vi "Lab Panel V5.25.vi"() -> ()   [LabVIEW 2017] (continued)
                        n1485 = stacked-sequence {
                          tunnel: w2788 -> [w2791 _]
                          tunnel: w2787 -> [_ w2796]
                          tunnel: w2786 -> [w2789 _]
                          frame #0 {
                            n1486 = Build Array("T-RISE") -> (w2793:string[])
                            n1487 = Build Array(w2791) -> (w2792:dbl[])
                            n1488 = TDMS Write(0:w2789, 5:"TEST PASS", 7:w2793, 9:w2792) -> (15:w2795:errorcluster)  [unwired: 2 in, 3 out]
                            n1489 = local write "data file error"(w2795) -> ()
                          }
                          frame #1 {
                            n1490 = Bundle(cluster=w2796, "STATUS"="T-RISE PASS") -> (w2798:T4)  [unwired: 2 in]
                            n1491 = local write "RESULT LAB05-1"(TRUE) -> ()
                            n1492 = local write "DISP LAB05-1"(w2798) -> ()
                          }
                        }
                      }
                      frame False {
                      }
                    }
                  }
                }
              }
              frame #9 {
                # "LAB05-2"
                n1493 = Equal?(x=w2801, y=2) -> (x = y?=w2804:bool)
                n1494 = local read "DISP LAB05-2"() -> (w2806:T4)
                n1495 = Unbundle(w2806) -> ("STATUS"=w2807:string)  [unwired: 2 out]
                n1496 = Equal?(x=w2807, y="RUN") -> (x = y?=w2803:bool)
                n1497 = And(x=w2803, y=w2804) -> (x .and. y?=w2802:bool)
                n1498 = case shown="True" w2802 {
                  tunnel: w2806 -> [_ w2810]
                  tunnel: w2800 -> [_ w2813]
                  frame False {
                  }
                  frame True {
                    n1499 = local read "SET LAB05-2"() -> (w2812:T5)
                    n1500 = local read "TDMS LAB05-2"() -> (w2809:refnum<k34>)
                    n1501 = Unbundle(w2810) -> ("CYCLE"=w2814:dbl)  [unwired: 2 out]
                    n1502 = Unbundle(w2812) -> ("T-RISE mins"=w2811:dbl)  [unwired: 4 out]
                    n1503 = Greater Or Equal?(x=w2814, y=w2813) -> (x >= y?=w2815:bool)
                    n1504 = case shown="True" w2815 {
                      tunnel: w2811 -> [w2818 _]
                      tunnel: w2810 -> [w2817 _]
                      tunnel: w2809 -> [w2816 _]
                      frame True {
                        n1505 = stacked-sequence {
                          tunnel: w2818 -> [w2821 _]
                          tunnel: w2817 -> [_ w2826]
                          tunnel: w2816 -> [w2819 _]
                          frame #0 {
                            n1506 = Build Array("T-RISE") -> (w2823:string[])
                            n1507 = Build Array(w2821) -> (w2822:dbl[])
                            n1508 = TDMS Write(0:w2819, 5:"TEST PASS", 7:w2823, 9:w2822) -> (15:w2825:errorcluster)  [unwired: 2 in, 3 out]
                            n1509 = local write "data file error"(w2825) -> ()
                          }
                          frame #1 {
                            n1510 = Bundle(cluster=w2826, "STATUS"="T-RISE PASS") -> (w2828:T4)  [unwired: 2 in]
                            n1511 = local write "RESULT LAB05-2"(TRUE) -> ()
                            n1512 = local write "DISP LAB05-2"(w2828) -> ()
                          }
                        }
                      }
                      frame False {
                      }
                    }
                  }
                }
              }
            }
          }
          frame #6 {
            # "end test & close test files"
            n1513 = local read "MAIL SETTINGS"() -> (w2834:T7)
            n1514 = Unbundle(w2834) -> ("OUT SERVER ADDRESS"=w2833:string, "FROM ACCOUNT"=w2832:string)  [unwired: 5 out]
            n1515 = stacked-sequence {
              tunnel: w2844 -> [_ _ _ _ _ _ _ _ _ _]
              tunnel: w2845 -> [_ _ _ _ _ _ _ _ _ _]
              tunnel: w2843 -> [_ _ _ _ _ _ _ _ _ _]
              tunnel: w2842 -> [_ _ _ _ _ _ _ _ _ _]
              tunnel: w2841 -> [_ _ _ _ _ _ _ _ _ _]
              tunnel: w2840 -> [_ _ _ _ _ _ _ _ _ _]
              tunnel: w2839 -> [_ _ _ _ _ _ _ _ _ _]
              tunnel: w2838 -> [_ _ _ _ _ _ _ _ _ _]
              tunnel: w2837 -> [_ _ _ _ _ _ _ _ _ _]
              tunnel: w2836 -> [_ _ _ _ _ _ _ _ _ _]
              tunnel: w2833 -> [w2849 w2901 w2949 w2996 w3043 w3090 w3137 w3184 w3231 w3278]
              tunnel: w2832 -> [w2848 w2900 w2948 w2995 w3042 w3089 w3136 w3183 w3230 w3277]
              tunnel: "Mail Test File To:" -> [w2847 w2899 w2947 w2994 w3041 w3088 w3135 w3182 w3229 w3276]
              tunnel: "Mail Test Fail" -> [w2846 w2898 w2946 w2993 w3040 w3087 w3134 w3181 w3228 w3275]
              frame #0 {
                # "LAB01-1"
                n1516 = local read "DISP LAB01-1"() -> (w2853:T4)
                n1517 = local read "run lab01-1"() -> (w2850:bool)
                n1518 = local read "TDMS LAB01-1"() -> (w2851:refnum<k34>)
                n1519 = Unbundle(w2853) -> ("CYCLE"=w2854:dbl, "STATUS"=w2852:string)  [unwired: 1 out]
                n1520 = case shown="True" w2850 {
                  tunnel: w2854 -> [_ w2860]
                  tunnel: w2853 -> [_ w2862]
                  tunnel: w2852 -> [_ w2859]
                  tunnel: w2851 -> [_ w2861]
                  tunnel: w2849 -> [_ w2858]
                  tunnel: w2848 -> [_ w2857]
                  tunnel: w2847 -> [_ w2856]
                  tunnel: w2846 -> [_ w2855]
                  frame False {
                  }
                  frame True {
                    n1521 = Not Equal?(x=w2859, y="RUN") -> (x != y?=w2863:bool)
                    n1522 = Greater?(x=w2860, y=2.0) -> (0:w2865:bool)
                    n1523 = And(x=w2865, y=w2863) -> (x .and. y?=w2864:bool)
                    n1524 = case shown="True" w2864 {
                      tunnel: w2862 -> [_ w2875]
                      tunnel: w2861 -> [_ w2874]
                      tunnel: w2860 -> [_ w2873]
                      tunnel: w2859 -> [_ w2872]
                      tunnel: w2858 -> [_ w2871]
                      tunnel: w2857 -> [_ w2870]
                      tunnel: w2856 -> [_ w2869]
                      tunnel: w2855 -> [_ w2868]
                      frame False {
                      }
                      frame True {
                        n1525 = stacked-sequence {
                          tunnel: w2875 -> [w2879 _ _]
                          tunnel: w2874 -> [_ w2881 _]
                          tunnel: w2873 -> [_ _ _]
                          tunnel: w2872 -> [_ _ w2887]
                          tunnel: w2871 -> [_ _ w2886]
                          tunnel: w2870 -> [_ _ w2885]
                          tunnel: w2869 -> [_ _ w2884]
                          tunnel: w2868 -> [_ _ w2883]
                          frame #0 {
                            w2876 = FALSE
                            n1526 = local write "mail control"("END") -> ()
                            n1527 = Bundle(cluster=w2879) -> (w2878:T4)  [unwired: 3 in]
                            n1528 = local write "DISP LAB01-1"(w2878) -> ()
                            n1529 = local write "O/I  LAB01-1"(w2876) -> ()
                            n1530 = local write "run lab01-1"(w2876) -> ()
                            n1531 = local write "RUN LAB01-1"(w2876) -> ()
                          }
                          frame #1 {
                            n1532 = TDMS Close(11:w2881) -> (0:w2880:errorcluster)  [unwired: 1 in, 1 out]
                            n1533 = local write "data file error"(w2880) -> ()
                          }
                          frame #2 {
                            n1534 = stacked-sequence {
                              tunnel: "LAB01-1" -> [w2889 w2891 _]
                              tunnel: w2887 -> [_ w2897 _]
                              tunnel: w2886 -> [_ w2896 _]
                              tunnel: w2885 -> [_ w2895 _]
                              tunnel: w2884 -> [_ w2894 _]
                              tunnel: w2883 -> [_ w2893 _]
                              frame #0 {
                                n1535 = call "sub vi - defrag tdms v1.vi"("panel id"=w2889) -> ("error out"=w2888:errorcluster)  [unwired: 10 in]
                                n1536 = local write "data file error"(w2888) -> ()
                              }
                              frame #1 {
                                n1537 = Bundle("STATUS"=w2897, "OUT SERVER ADDRESS"=w2896, "FROM ACCOUNT"=w2895, "Mail Test File To:"=w2894, "Mail Test Fail"=w2893) -> (w2890:T26)  [unwired: 1 in]
                                n1538 = call "Save data file (pass-fail) v5.vi"("Input Cluster"=w2890, "panel id"=w2891) -> ("network file save error"=w2892:errorcluster)  [unwired: 8 in, 1 out]
                                n1539 = local write "data file error"(w2892) -> ()
                              }
                              frame #2 {
                              }
                            }
                          }
                        }
                      }
                    }
                  }
                }
              }
              frame #1 {
                # "LAB01-2"
                n1540 = local read "run lab01-2"() -> (w2902:bool)
                n1541 = case shown="True" w2902 {
                  tunnel: w2901 -> [_ w2906]
                  tunnel: w2900 -> [_ w2905]
                  tunnel: w2899 -> [_ w2904]
                  tunnel: w2898 -> [_ w2903]
                  frame False {
                  }
                  frame True {
                    n1542 = local read "DISP LAB01-2"() -> (w2914:T4)
                    n1543 = local read "TDMS LAB01-2"() -> (w2913:refnum<k34>)
                    n1544 = Unbundle(w2914) -> ("CYCLE"=w2908:dbl, "STATUS"=w2907:string)  [unwired: 1 out]
                    n1545 = Not Equal?(x=w2907, y="RUN") -> (x != y?=w2910:bool)
                    n1546 = Greater?(x=w2908, y=2.0) -> (0:w2911:bool)
                    n1547 = And(x=w2911, y=w2910) -> (x .and. y?=w2909:bool)
                    n1548 = case shown="True" w2909 {
                      tunnel: w2914 -> [_ w2923]
                      tunnel: w2913 -> [_ w2922]
                      tunnel: w2908 -> [_ w2921]
                      tunnel: w2907 -> [_ w2920]
                      tunnel: w2906 -> [_ w2919]
                      tunnel: w2905 -> [_ w2918]
                      tunnel: w2904 -> [_ w2917]
                      tunnel: w2903 -> [_ w2916]
                      frame False {
                      }
                      frame True {
                        n1549 = stacked-sequence {
                          tunnel: w2923 -> [w2926 _ _]
                          tunnel: w2922 -> [_ w2928 _]
                          tunnel: w2921 -> [_ _ _]
                          tunnel: w2920 -> [_ _ w2934]
                          tunnel: w2919 -> [_ _ w2933]
                          tunnel: w2918 -> [_ _ w2932]
                          tunnel: w2917 -> [_ _ w2931]
                          tunnel: w2916 -> [_ _ w2930]
                          frame #0 {
                            w2924 = FALSE
                            n1550 = local write "mail control"("END") -> ()
                            n1551 = Bundle(cluster=w2926) -> (w2927:T4)  [unwired: 3 in]
                            n1552 = local write "RUN LAB01-2"(w2924) -> ()
                            n1553 = local write "run lab01-2"(w2924) -> ()
                            n1554 = local write "O/I  LAB01-2"(w2924) -> ()
                            n1555 = local write "DISP LAB01-2"(w2927) -> ()
                          }
                          frame #1 {
                            n1556 = TDMS Close(11:w2928) -> (0:w2929:errorcluster)  [unwired: 1 in, 1 out]
                            n1557 = local write "data file error"(w2929) -> ()
                          }
                          frame #2 {
                            n1558 = stacked-sequence {
                              tunnel: "LAB01-2" -> [w2937 w2938]
                              tunnel: w2934 -> [_ w2943]
                              tunnel: w2933 -> [_ w2942]
                              tunnel: w2932 -> [_ w2941]
                              tunnel: w2931 -> [_ w2940]
                              tunnel: w2930 -> [_ w2939]
                              frame #0 {
                                n1559 = call "sub vi - defrag tdms v1.vi"("panel id"=w2937) -> ("error out"=w2936:errorcluster)  [unwired: 10 in]
                                n1560 = local write "data file error"(w2936) -> ()
                              }
                              frame #1 {
                                n1561 = Bundle("STATUS"=w2943, "OUT SERVER ADDRESS"=w2942, "FROM ACCOUNT"=w2941, "Mail Test File To:"=w2940, "Mail Test Fail"=w2939) -> (w2945:T26)  [unwired: 1 in]
                                n1562 = call "Save data file (pass-fail) v5.vi"("Input Cluster"=w2945, "panel id"=w2938) -> ("network file save error"=w2944:errorcluster)  [unwired: 8 in, 1 out]
                                n1563 = local write "data file error"(w2944) -> ()
                              }
                            }
                          }
                        }
                      }
                    }
                  }
                }
              }
              frame #2 {
                # "LAB02-1"
                n1564 = local read "run lab02-1"() -> (w2950:bool)
                n1565 = case shown="True" w2950 {
                  tunnel: w2949 -> [_ w2954]
                  tunnel: w2948 -> [_ w2953]
                  tunnel: w2947 -> [_ w2952]
                  tunnel: w2946 -> [_ w2951]
                  frame False {
                  }
                  frame True {
                    n1566 = local read "DISP LAB02-1"() -> (w2962:T4)
                    n1567 = Unbundle(w2962) -> ("CYCLE"=w2958:dbl, "STATUS"=w2955:string)  [unwired: 1 out]
                    n1568 = local read "TDMS LAB02-1"() -> (w2961:refnum<k34>)
                    n1569 = Not Equal?(x=w2955, y="RUN") -> (x != y?=w2957:bool)
                    n1570 = Greater?(x=w2958, y=2.0) -> (0:w2959:bool)
                    n1571 = And(x=w2959, y=w2957) -> (x .and. y?=w2956:bool)
                    n1572 = case shown="True" w2956 {
                      tunnel: w2962 -> [_ w2970]
                      tunnel: w2961 -> [_ w2969]
                      tunnel: w2955 -> [_ w2968]
                      tunnel: w2954 -> [_ w2967]
                      tunnel: w2953 -> [_ w2966]
                      tunnel: w2952 -> [_ w2965]
                      tunnel: w2951 -> [_ w2964]
                      frame False {
                      }
                      frame True {
                        n1573 = stacked-sequence {
                          tunnel: w2970 -> [w2973 _ _]
                          tunnel: w2969 -> [_ w2975 _]
                          tunnel: w2968 -> [_ _ w2981]
                          tunnel: w2967 -> [_ _ w2980]
                          tunnel: w2966 -> [_ _ w2979]
                          tunnel: w2965 -> [_ _ w2978]
                          tunnel: w2964 -> [_ _ w2977]
                          frame #0 {
                            w2971 = FALSE
                            n1574 = local write "mail control"("END") -> ()
                            n1575 = Bundle(cluster=w2973) -> (w2974:T4)  [unwired: 3 in]
                            n1576 = local write "O/I  LAB02-1"(w2971) -> ()
                            n1577 = local write "RUN LAB02-1"(w2971) -> ()
                            n1578 = local write "run lab02-1"(w2971) -> ()
                            n1579 = local write "DISP LAB02-1"(w2974) -> ()
                          }
                          frame #1 {
                            n1580 = TDMS Close(11:w2975) -> (0:w2976:errorcluster)  [unwired: 1 in, 1 out]
                            n1581 = local write "data file error"(w2976) -> ()
                          }
                          frame #2 {
                            n1582 = stacked-sequence {
                              tunnel: "LAB02-1" -> [w2984 w2991]
                              tunnel: w2981 -> [_ w2989]
                              tunnel: w2980 -> [_ w2988]
                              tunnel: w2979 -> [_ w2987]
                              tunnel: w2978 -> [_ w2986]
                              tunnel: w2977 -> [_ w2985]
                              frame #0 {
                                n1583 = call "sub vi - defrag tdms v1.vi"("panel id"=w2984) -> ("error out"=w2983:errorcluster)  [unwired: 10 in]
                                n1584 = local write "data file error"(w2983) -> ()
                              }
                              frame #1 {
                                n1585 = Bundle("STATUS"=w2989, "OUT SERVER ADDRESS"=w2988, "FROM ACCOUNT"=w2987, "Mail Test File To:"=w2986, "Mail Test Fail"=w2985) -> (w2990:T26)  [unwired: 1 in]
                                n1586 = call "Save data file (pass-fail) v5.vi"("Input Cluster"=w2990, "panel id"=w2991) -> ("network file save error"=w2992:errorcluster)  [unwired: 8 in, 1 out]
                                n1587 = local write "data file error"(w2992) -> ()
                              }
                            }
                          }
                        }
                      }
                    }
                  }
                }
              }
              frame #3 {
                # "LAB02-2"
                n1588 = local read "run lab02-2"() -> (w2997:bool)
                n1589 = case shown="True" w2997 {
                  tunnel: w2996 -> [_ w3001]
                  tunnel: w2995 -> [_ w3000]
                  tunnel: w2994 -> [_ w2999]
                  tunnel: w2993 -> [_ w2998]
                  frame False {
                  }
                  frame True {
                    n1590 = local read "DISP LAB02-2"() -> (w3009:T4)
                    n1591 = local read "TDMS LAB02-2"() -> (w3008:refnum<k34>)
                    n1592 = Unbundle(w3009) -> ("CYCLE"=w3005:dbl, "STATUS"=w3002:string)  [unwired: 1 out]
                    n1593 = Not Equal?(x=w3002, y="RUN") -> (x != y?=w3004:bool)
                    n1594 = Greater?(x=w3005, y=2.0) -> (0:w3006:bool)
                    n1595 = And(x=w3006, y=w3004) -> (x .and. y?=w3003:bool)
                    n1596 = case shown="True" w3003 {
                      tunnel: w3009 -> [_ w3017]
                      tunnel: w3008 -> [_ w3016]
                      tunnel: w3002 -> [_ w3015]
                      tunnel: w3001 -> [_ w3014]
                      tunnel: w3000 -> [_ w3013]
                      tunnel: w2999 -> [_ w3012]
                      tunnel: w2998 -> [_ w3011]
                      frame False {
                      }
                      frame True {
                        n1597 = stacked-sequence {
                          tunnel: w3017 -> [w3020 _ _]
                          tunnel: w3016 -> [_ w3022 _]
                          tunnel: w3015 -> [_ _ w3028]
                          tunnel: w3014 -> [_ _ w3027]
                          tunnel: w3013 -> [_ _ w3026]
                          tunnel: w3012 -> [_ _ w3025]
                          tunnel: w3011 -> [_ _ w3024]
                          frame #0 {
                            w3018 = FALSE
                            n1598 = local write "mail control"("END") -> ()
                            n1599 = Bundle(cluster=w3020) -> (w3021:T4)  [unwired: 3 in]
                            n1600 = local write "O/I  LAB02-2"(w3018) -> ()
                            n1601 = local write "run lab02-2"(w3018) -> ()
                            n1602 = local write "RUN LAB02-2"(w3018) -> ()
                            n1603 = local write "DISP LAB02-2"(w3021) -> ()
                          }
                          frame #1 {
                            n1604 = TDMS Close(11:w3022) -> (0:w3023:errorcluster)  [unwired: 1 in, 1 out]
                            n1605 = local write "data file error"(w3023) -> ()
                          }
                          frame #2 {
                            n1606 = stacked-sequence {
                              tunnel: "LAB02-2" -> [w3031 w3037]
                              tunnel: w3028 -> [_ w3036]
                              tunnel: w3027 -> [_ w3035]
                              tunnel: w3026 -> [_ w3034]
                              tunnel: w3025 -> [_ w3033]
                              tunnel: w3024 -> [_ w3032]
                              frame #0 {
                                n1607 = call "sub vi - defrag tdms v1.vi"("panel id"=w3031) -> ("error out"=w3030:errorcluster)  [unwired: 10 in]
                                n1608 = local write "data file error"(w3030) -> ()
                              }
                              frame #1 {
                                n1609 = Bundle("STATUS"=w3036, "OUT SERVER ADDRESS"=w3035, "FROM ACCOUNT"=w3034, "Mail Test File To:"=w3033, "Mail Test Fail"=w3032) -> (w3039:T26)  [unwired: 1 in]
                                n1610 = call "Save data file (pass-fail) v5.vi"("Input Cluster"=w3039, "panel id"=w3037) -> ("network file save error"=w3038:errorcluster)  [unwired: 8 in, 1 out]
                                n1611 = local write "data file error"(w3038) -> ()
                              }
                            }
                          }
                        }
                      }
                    }
                  }
                }
              }
              frame #4 {
                # "LAB03-1"
                n1612 = local read "run lab03-1"() -> (w3044:bool)
                n1613 = case shown="True" w3044 {
                  tunnel: w3043 -> [_ w3048]
                  tunnel: w3042 -> [_ w3047]
                  tunnel: w3041 -> [_ w3046]
                  tunnel: w3040 -> [_ w3045]
                  frame False {
                  }
                  frame True {
                    n1614 = local read "DISP LAB03-1"() -> (w3056:T4)
                    n1615 = local read "TDMS LAB03-1"() -> (w3055:refnum<k34>)
                    n1616 = Unbundle(w3056) -> ("CYCLE"=w3052:dbl, "STATUS"=w3049:string)  [unwired: 1 out]
                    n1617 = Not Equal?(x=w3049, y="RUN") -> (x != y?=w3051:bool)
                    n1618 = Greater?(x=w3052, y=2.0) -> (0:w3053:bool)
                    n1619 = And(x=w3053, y=w3051) -> (x .and. y?=w3050:bool)
                    n1620 = case shown="True" w3050 {
                      tunnel: w3056 -> [_ w3064]
                      tunnel: w3055 -> [_ w3063]
                      tunnel: w3049 -> [_ w3062]
                      tunnel: w3048 -> [_ w3061]
                      tunnel: w3047 -> [_ w3060]
                      tunnel: w3046 -> [_ w3059]
                      tunnel: w3045 -> [_ w3058]
                      frame False {
                      }
                      frame True {
                        n1621 = stacked-sequence {
                          tunnel: w3064 -> [w3067 _ _]
                          tunnel: w3063 -> [_ w3069 _]
                          tunnel: w3062 -> [_ _ w3075]
                          tunnel: w3061 -> [_ _ w3074]
                          tunnel: w3060 -> [_ _ w3073]
                          tunnel: w3059 -> [_ _ w3072]
                          tunnel: w3058 -> [_ _ w3071]
                          frame #0 {
                            w3065 = FALSE
                            n1622 = local write "mail control"("END") -> ()
                            n1623 = Bundle(cluster=w3067) -> (w3068:T4)  [unwired: 3 in]
                            n1624 = local write "O/I  LAB03-1"(w3065) -> ()
                            n1625 = local write "run lab03-1"(w3065) -> ()
                            n1626 = local write "RUN LAB03-1"(w3065) -> ()
                            n1627 = local write "DISP LAB03-1"(w3068) -> ()
                          }
                          frame #1 {
                            n1628 = TDMS Close(11:w3069) -> (0:w3070:errorcluster)  [unwired: 1 in, 1 out]
                            n1629 = local write "data file error"(w3070) -> ()
                          }
                          frame #2 {
                            n1630 = stacked-sequence {
                              tunnel: "LAB03-1" -> [w3078 w3084]
                              tunnel: w3075 -> [_ w3083]
                              tunnel: w3074 -> [_ w3082]
                              tunnel: w3073 -> [_ w3081]
                              tunnel: w3072 -> [_ w3080]
                              tunnel: w3071 -> [_ w3079]
                              frame #0 {
                                n1631 = call "sub vi - defrag tdms v1.vi"("panel id"=w3078) -> ("error out"=w3077:errorcluster)  [unwired: 10 in]
                                n1632 = local write "data file error"(w3077) -> ()
                              }
                              frame #1 {
                                n1633 = Bundle("STATUS"=w3083, "OUT SERVER ADDRESS"=w3082, "FROM ACCOUNT"=w3081, "Mail Test File To:"=w3080, "Mail Test Fail"=w3079) -> (w3086:T26)  [unwired: 1 in]
                                n1634 = call "Save data file (pass-fail) v5.vi"("Input Cluster"=w3086, "panel id"=w3084) -> ("network file save error"=w3085:errorcluster)  [unwired: 8 in, 1 out]
                                n1635 = local write "data file error"(w3085) -> ()
                              }
                            }
                          }
                        }
                      }
                    }
                  }
                }
              }
              frame #5 {
                # "LAB03-2"
                n1636 = local read "run lab03-2"() -> (w3091:bool)
                n1637 = case shown="True" w3091 {
                  tunnel: w3090 -> [_ w3095]
                  tunnel: w3089 -> [_ w3094]
                  tunnel: w3088 -> [_ w3093]
                  tunnel: w3087 -> [_ w3092]
                  frame False {
                  }
                  frame True {
                    n1638 = local read "DISP LAB03-2"() -> (w3103:T4)
                    n1639 = Unbundle(w3103) -> ("CYCLE"=w3099:dbl, "STATUS"=w3096:string)  [unwired: 1 out]
                    n1640 = local read "TDMS LAB03-2"() -> (w3102:refnum<k34>)
                    n1641 = Not Equal?(x=w3096, y="RUN") -> (x != y?=w3098:bool)
                    n1642 = Greater?(x=w3099, y=2.0) -> (0:w3100:bool)
                    n1643 = And(x=w3100, y=w3098) -> (x .and. y?=w3097:bool)
                    n1644 = case shown="True" w3097 {
                      tunnel: w3103 -> [_ w3111]
                      tunnel: w3102 -> [_ w3110]
                      tunnel: w3096 -> [_ w3109]
                      tunnel: w3095 -> [_ w3108]
                      tunnel: w3094 -> [_ w3107]
                      tunnel: w3093 -> [_ w3106]
                      tunnel: w3092 -> [_ w3105]
                      frame False {
                      }
                      frame True {
                        n1645 = stacked-sequence {
                          tunnel: w3111 -> [w3114 _ _]
                          tunnel: w3110 -> [_ w3116 _]
                          tunnel: w3109 -> [_ _ w3122]
                          tunnel: w3108 -> [_ _ w3121]
                          tunnel: w3107 -> [_ _ w3120]
                          tunnel: w3106 -> [_ _ w3119]
                          tunnel: w3105 -> [_ _ w3118]
                          frame #0 {
                            w3112 = FALSE
                            n1646 = local write "mail control"("END") -> ()
                            n1647 = Bundle(cluster=w3114) -> (w3115:T4)  [unwired: 3 in]
                            n1648 = local write "RUN LAB03-2"(w3112) -> ()
                            n1649 = local write "O/I  LAB03-2"(w3112) -> ()
                            n1650 = local write "DISP LAB03-2"(w3115) -> ()
                            n1651 = local write "run lab03-2"(w3112) -> ()
                          }
                          frame #1 {
                            n1652 = TDMS Close(11:w3116) -> (0:w3117:errorcluster)  [unwired: 1 in, 1 out]
                            n1653 = local write "data file error"(w3117) -> ()
                          }
                          frame #2 {
                            n1654 = stacked-sequence {
                              tunnel: "LAB03-2" -> [w3125 w3126]
                              tunnel: w3122 -> [_ w3131]
                              tunnel: w3121 -> [_ w3130]
                              tunnel: w3120 -> [_ w3129]
                              tunnel: w3119 -> [_ w3128]
                              tunnel: w3118 -> [_ w3127]
                              frame #0 {
                                n1655 = call "sub vi - defrag tdms v1.vi"("panel id"=w3125) -> ("error out"=w3124:errorcluster)  [unwired: 10 in]
                                n1656 = local write "data file error"(w3124) -> ()
                              }
                              frame #1 {
                                n1657 = Bundle("STATUS"=w3131, "OUT SERVER ADDRESS"=w3130, "FROM ACCOUNT"=w3129, "Mail Test File To:"=w3128, "Mail Test Fail"=w3127) -> (w3133:T26)  [unwired: 1 in]
                                n1658 = call "Save data file (pass-fail) v5.vi"("Input Cluster"=w3133, "panel id"=w3126) -> ("network file save error"=w3132:errorcluster)  [unwired: 8 in, 1 out]
                                n1659 = local write "data file error"(w3132) -> ()
                              }
                            }
                          }
                        }
                      }
                    }
                  }
                }
              }
              frame #6 {
                # "LAB04-1"
                n1660 = local read "run lab04-1"() -> (w3138:bool)
                n1661 = case shown="True" w3138 {
                  tunnel: w3137 -> [_ w3142]
                  tunnel: w3136 -> [_ w3141]
                  tunnel: w3135 -> [_ w3140]
                  tunnel: w3134 -> [_ w3139]
                  frame False {
                  }
                  frame True {
                    n1662 = local read "DISP LAB04-1"() -> (w3150:T4)
                    n1663 = Unbundle(w3150) -> ("CYCLE"=w3146:dbl, "STATUS"=w3143:string)  [unwired: 1 out]
                    n1664 = local read "TDMS LAB04-1"() -> (w3149:refnum<k34>)
                    n1665 = Not Equal?(x=w3143, y="RUN") -> (x != y?=w3145:bool)
                    n1666 = Greater?(x=w3146, y=2.0) -> (0:w3147:bool)
                    n1667 = And(x=w3147, y=w3145) -> (x .and. y?=w3144:bool)
                    n1668 = case shown="True" w3144 {
                      tunnel: w3150 -> [_ w3158]
                      tunnel: w3149 -> [_ w3157]
                      tunnel: w3143 -> [_ w3156]
                      tunnel: w3142 -> [_ w3155]
                      tunnel: w3141 -> [_ w3154]
                      tunnel: w3140 -> [_ w3153]
                      tunnel: w3139 -> [_ w3152]
                      frame False {
                      }
                      frame True {
                        n1669 = stacked-sequence {
                          tunnel: w3158 -> [w3161 _ _]
                          tunnel: w3157 -> [_ w3163 _]
                          tunnel: w3156 -> [_ _ w3169]
                          tunnel: w3155 -> [_ _ w3168]
                          tunnel: w3154 -> [_ _ w3167]
                          tunnel: w3153 -> [_ _ w3166]
                          tunnel: w3152 -> [_ _ w3165]
                          frame #0 {
                            w3159 = FALSE
                            n1670 = local write "mail control"("END") -> ()
                            n1671 = Bundle(cluster=w3161) -> (w3162:T4)  [unwired: 3 in]
                            n1672 = local write "RUN LAB04-1"(w3159) -> ()
                            n1673 = local write "O/I  LAB04-1"(w3159) -> ()
                            n1674 = local write "run lab04-1"(w3159) -> ()
                            n1675 = local write "DISP LAB04-1"(w3162) -> ()
                          }
                          frame #1 {
                            n1676 = TDMS Close(11:w3163) -> (0:w3164:errorcluster)  [unwired: 1 in, 1 out]
                            n1677 = local write "data file error"(w3164) -> ()
                          }
                          frame #2 {
                            n1678 = stacked-sequence {
                              tunnel: "LAB04-1" -> [w3172 w3173]
                              tunnel: w3169 -> [_ w3178]
                              tunnel: w3168 -> [_ w3177]
                              tunnel: w3167 -> [_ w3176]
                              tunnel: w3166 -> [_ w3175]
                              tunnel: w3165 -> [_ w3174]
                              frame #0 {
                                n1679 = call "sub vi - defrag tdms v1.vi"("panel id"=w3172) -> ("error out"=w3171:errorcluster)  [unwired: 10 in]
                                n1680 = local write "data file error"(w3171) -> ()
                              }
                              frame #1 {
                                n1681 = Bundle("STATUS"=w3178, "OUT SERVER ADDRESS"=w3177, "FROM ACCOUNT"=w3176, "Mail Test File To:"=w3175, "Mail Test Fail"=w3174) -> (w3180:T26)  [unwired: 1 in]
                                n1682 = call "Save data file (pass-fail) v5.vi"("Input Cluster"=w3180, "panel id"=w3173) -> ("network file save error"=w3179:errorcluster)  [unwired: 8 in, 1 out]
                                n1683 = local write "data file error"(w3179) -> ()
                              }
                            }
                          }
                        }
                      }
                    }
                  }
                }
              }
              frame #7 {
                # "LAB04-2"
                n1684 = local read "run lab04-2"() -> (w3185:bool)
                n1685 = case shown="True" w3185 {
                  tunnel: w3184 -> [_ w3189]
                  tunnel: w3183 -> [_ w3188]
                  tunnel: w3182 -> [_ w3187]
                  tunnel: w3181 -> [_ w3186]
                  frame False {
                  }
                  frame True {
                    n1686 = local read "DISP LAB04-2"() -> (w3197:T4)
                    n1687 = Unbundle(w3197) -> ("CYCLE"=w3193:dbl, "STATUS"=w3190:string)  [unwired: 1 out]
                    n1688 = Not Equal?(x=w3190, y="RUN") -> (x != y?=w3192:bool)
                    n1689 = local read "TDMS LAB04-2"() -> (w3196:refnum<k34>)
                    n1690 = Greater?(x=w3193, y=2.0) -> (0:w3194:bool)
                    n1691 = And(x=w3194, y=w3192) -> (x .and. y?=w3191:bool)
                    n1692 = case shown="True" w3191 {
                      tunnel: w3197 -> [_ w3205]
                      tunnel: w3196 -> [_ w3204]
                      tunnel: w3190 -> [_ w3203]
                      tunnel: w3189 -> [_ w3202]
                      tunnel: w3188 -> [_ w3201]
                      tunnel: w3187 -> [_ w3200]
                      tunnel: w3186 -> [_ w3199]
                      frame False {
                      }
                      frame True {
                        n1693 = stacked-sequence {
                          tunnel: w3205 -> [w3208 _ _]
                          tunnel: w3204 -> [_ w3210 _]
                          tunnel: w3203 -> [_ _ w3216]
                          tunnel: w3202 -> [_ _ w3215]
                          tunnel: w3201 -> [_ _ w3214]
                          tunnel: w3200 -> [_ _ w3213]
                          tunnel: w3199 -> [_ _ w3212]
                          frame #0 {
                            w3206 = FALSE
                            n1694 = local write "mail control"("END") -> ()
                            n1695 = Bundle(cluster=w3208) -> (w3209:T4)  [unwired: 3 in]
                            n1696 = local write "O/I  LAB04-2"(w3206) -> ()
                            n1697 = local write "RUN LAB04-2"(w3206) -> ()
                            n1698 = local write "run lab04-2"(w3206) -> ()
                            n1699 = local write "DISP LAB04-2"(w3209) -> ()
                          }
                          frame #1 {
                            n1700 = TDMS Close(11:w3210) -> (0:w3211:errorcluster)  [unwired: 1 in, 1 out]
                            n1701 = local write "data file error"(w3211) -> ()
                          }
                          frame #2 {
                            n1702 = stacked-sequence {
                              tunnel: "LAB04-2" -> [w3219 w3220]
                              tunnel: w3216 -> [_ w3225]
                              tunnel: w3215 -> [_ w3224]
                              tunnel: w3214 -> [_ w3223]
                              tunnel: w3213 -> [_ w3222]
                              tunnel: w3212 -> [_ w3221]
                              frame #0 {
                                n1703 = call "sub vi - defrag tdms v1.vi"("panel id"=w3219) -> ("error out"=w3218:errorcluster)  [unwired: 10 in]
                                n1704 = local write "data file error"(w3218) -> ()
                              }
                              frame #1 {
                                n1705 = Bundle("STATUS"=w3225, "OUT SERVER ADDRESS"=w3224, "FROM ACCOUNT"=w3223, "Mail Test File To:"=w3222, "Mail Test Fail"=w3221) -> (w3227:T26)  [unwired: 1 in]
                                n1706 = call "Save data file (pass-fail) v5.vi"("Input Cluster"=w3227, "panel id"=w3220) -> ("network file save error"=w3226:errorcluster)  [unwired: 8 in, 1 out]
                                n1707 = local write "data file error"(w3226) -> ()
                              }
                            }
                          }
                        }
                      }
                    }
                  }
                }
              }
              frame #8 {
                # "LAB05-1"
                n1708 = local read "run lab05-1"() -> (w3232:bool)
                n1709 = case shown="True" w3232 {
                  tunnel: w3231 -> [_ w3236]
                  tunnel: w3230 -> [_ w3235]
                  tunnel: w3229 -> [_ w3234]
                  tunnel: w3228 -> [_ w3233]
                  frame False {
                  }
                  frame True {
                    n1710 = local read "DISP LAB05-1"() -> (w3244:T4)
                    n1711 = Unbundle(w3244) -> ("CYCLE"=w3240:dbl, "STATUS"=w3237:string)  [unwired: 1 out]
                    n1712 = Not Equal?(x=w3237, y="RUN") -> (x != y?=w3239:bool)
                    n1713 = local read "TDMS LAB05-1"() -> (w3243:refnum<k34>)
                    n1714 = Greater?(x=w3240, y=2.0) -> (0:w3241:bool)
                    n1715 = And(x=w3241, y=w3239) -> (x .and. y?=w3238:bool)
                    n1716 = case shown="True" w3238 {
                      tunnel: w3244 -> [_ w3252]
                      tunnel: w3243 -> [_ w3251]
                      tunnel: w3237 -> [_ w3250]
                      tunnel: w3236 -> [_ w3249]
                      tunnel: w3235 -> [_ w3248]
                      tunnel: w3234 -> [_ w3247]
                      tunnel: w3233 -> [_ w3246]
                      frame False {
                      }
                      frame True {
                        n1717 = stacked-sequence {
                          tunnel: w3252 -> [w3255 _ _]
                          tunnel: w3251 -> [_ w3257 _]
                          tunnel: w3250 -> [_ _ w3263]
                          tunnel: w3249 -> [_ _ w3262]
                          tunnel: w3248 -> [_ _ w3261]
                          tunnel: w3247 -> [_ _ w3260]
                          tunnel: w3246 -> [_ _ w3259]
                          frame #0 {
                            w3253 = FALSE
                            n1718 = local write "mail control"("END") -> ()
                            n1719 = Bundle(cluster=w3255) -> (w3256:T4)  [unwired: 3 in]
                            n1720 = local write "O/I  LAB05-1"(w3253) -> ()
                            n1721 = local write "RUN LAB05-1"(w3253) -> ()
                            n1722 = local write "run lab05-1"(w3253) -> ()
                            n1723 = local write "DISP LAB05-1"(w3256) -> ()
                          }
                          frame #1 {
                            n1724 = TDMS Close(11:w3257) -> (0:w3258:errorcluster)  [unwired: 1 in, 1 out]
                            n1725 = local write "data file error"(w3258) -> ()
                          }
                          frame #2 {
                            n1726 = stacked-sequence {
                              tunnel: "LAB05-1" -> [w3266 w3272]
                              tunnel: w3263 -> [_ w3271]
                              tunnel: w3262 -> [_ w3270]
                              tunnel: w3261 -> [_ w3269]
                              tunnel: w3260 -> [_ w3268]
                              tunnel: w3259 -> [_ w3267]
                              frame #0 {
                                n1727 = call "sub vi - defrag tdms v1.vi"("panel id"=w3266) -> ("error out"=w3265:errorcluster)  [unwired: 10 in]
                                n1728 = local write "data file error"(w3265) -> ()
                              }
                              frame #1 {
                                n1729 = Bundle("STATUS"=w3271, "OUT SERVER ADDRESS"=w3270, "FROM ACCOUNT"=w3269, "Mail Test File To:"=w3268, "Mail Test Fail"=w3267) -> (w3274:T26)  [unwired: 1 in]
                                n1730 = call "Save data file (pass-fail) v5.vi"("Input Cluster"=w3274, "panel id"=w3272) -> ("network file save error"=w3273:errorcluster)  [unwired: 8 in, 1 out]
                                n1731 = local write "data file error"(w3273) -> ()
                              }
                            }
                          }
                        }
                      }
                    }
                  }
                }
              }
              frame #9 {
                # "LAB05-2"
                n1732 = local read "run lab05-2"() -> (w3279:bool)
                n1733 = case shown="True" w3279 {
                  tunnel: w3278 -> [_ w3283]
                  tunnel: w3277 -> [_ w3282]
                  tunnel: w3276 -> [_ w3281]
                  tunnel: w3275 -> [_ w3280]
                  frame False {
                  }
                  frame True {
                    n1734 = local read "DISP LAB05-2"() -> (w3291:T4)
                    n1735 = Unbundle(w3291) -> ("CYCLE"=w3287:dbl, "STATUS"=w3284:string)  [unwired: 1 out]
                    n1736 = Not Equal?(x=w3284, y="RUN") -> (x != y?=w3286:bool)
                    n1737 = local read "TDMS LAB05-2"() -> (w3290:refnum<k34>)
                    n1738 = Greater?(x=w3287, y=2.0) -> (0:w3288:bool)
                    n1739 = And(x=w3288, y=w3286) -> (x .and. y?=w3285:bool)
                    n1740 = case shown="True" w3285 {
                      tunnel: w3291 -> [_ w3299]
                      tunnel: w3290 -> [_ w3298]
                      tunnel: w3284 -> [_ w3297]
                      tunnel: w3283 -> [_ w3296]
                      tunnel: w3282 -> [_ w3295]
                      tunnel: w3281 -> [_ w3294]
                      tunnel: w3280 -> [_ w3293]
                      frame False {
                      }
                      frame True {
                        n1741 = stacked-sequence {
                          tunnel: w3299 -> [w3302 _ _]
                          tunnel: w3298 -> [_ w3304 _]
                          tunnel: w3297 -> [_ _ w3310]
                          tunnel: w3296 -> [_ _ w3309]
                          tunnel: w3295 -> [_ _ w3308]
                          tunnel: w3294 -> [_ _ w3307]
                          tunnel: w3293 -> [_ _ w3306]
                          frame #0 {
                            w3300 = FALSE
                            n1742 = local write "mail control"("END") -> ()
                            n1743 = Bundle(cluster=w3302) -> (w3303:T4)  [unwired: 3 in]
                            n1744 = local write "RUN LAB05-2"(w3300) -> ()
                            n1745 = local write "O/I  LAB05-2"(w3300) -> ()
                            n1746 = local write "run lab05-2"(w3300) -> ()
                            n1747 = local write "DISP LAB05-2"(w3303) -> ()
                          }
                          frame #1 {
                            n1748 = TDMS Close(11:w3304) -> (0:w3305:errorcluster)  [unwired: 1 in, 1 out]
                            n1749 = local write "data file error"(w3305) -> ()
                          }
                          frame #2 {
                            n1750 = stacked-sequence {
                              tunnel: "LAB05-2" -> [w3313 w3319]
                              tunnel: w3310 -> [_ w3318]
                              tunnel: w3309 -> [_ w3317]
                              tunnel: w3308 -> [_ w3316]
                              tunnel: w3307 -> [_ w3315]
                              tunnel: w3306 -> [_ w3314]
                              frame #0 {
                                n1751 = call "sub vi - defrag tdms v1.vi"("panel id"=w3313) -> ("error out"=w3312:errorcluster)  [unwired: 10 in]
                                n1752 = local write "data file error"(w3312) -> ()
                              }
                              frame #1 {
                                n1753 = Bundle("STATUS"=w3318, "OUT SERVER ADDRESS"=w3317, "FROM ACCOUNT"=w3316, "Mail Test File To:"=w3315, "Mail Test Fail"=w3314) -> (w3321:T26)  [unwired: 1 in]
                                n1754 = call "Save data file (pass-fail) v5.vi"("Input Cluster"=w3321, "panel id"=w3319) -> ("network file save error"=w3320:errorcluster)  [unwired: 8 in, 1 out]
                                n1755 = local write "data file error"(w3320) -> ()
                              }
                            }
                          }
                        }
                      }
                    }
                  }
                }
              }
            }
            n1756 = local read "Network Directory"() -> (w2835:path)
            n1757 = global write "Global 1.vi" "Network Drive"(w2835) -> ()
          }
          frame #7 {
            # "disable functions"
            n1758 = stacked-sequence {
              tunnel: w3331 -> [w3345 _ w3402]
              tunnel: w3330 -> [w3340 _ w3401]
              tunnel: w3329 -> [w3339 _ w3400]
              tunnel: w3328 -> [w3337 _ w3399]
              tunnel: w3327 -> [w3338 _ w3398]
              tunnel: w3326 -> [_ w3362 w3397]
              tunnel: w3325 -> [_ w3363 w3396]
              tunnel: w3324 -> [_ w3364 w3395]
              tunnel: w3323 -> [_ w3365 w3394]
              tunnel: w3322 -> [_ w3366 w3393]
              frame #0 {
                n1759 = Select(t=2, s=w3337, f=0) -> (s? t:f=w3333:i32)
                n1760 = Select(t=2, s=w3339, f=0) -> (s? t:f=w3334:i32)
                n1761 = Select(t=2, s=w3338, f=0) -> (s? t:f=w3332:i32)
                n1762 = Select(t=2, s=w3345, f=0) -> (s? t:f=w3336:i32)
                n1763 = Select(t=2, s=w3340, f=0) -> (s? t:f=w3335:i32)
                n1764 = property on="SELECT LAB02-2" class="RadioBtnsControl (strict)"("DisabledEnum"=w3333) -> ()  [unwired: 2 in, 2 out]
                n1765 = property on="SELECT LAB02-1" class="RadioBtnsControl (strict)"("DisabledEnum"=w3334) -> ()  [unwired: 2 in, 2 out]
                n1766 = property on="SELECT LAB03-1" class="RadioBtnsControl (strict)"("DisabledEnum"=w3332) -> ()  [unwired: 2 in, 2 out]
                n1767 = property on="SELECT LAB01-1" class="RadioBtnsControl (strict)"("DisabledEnum"=w3336) -> ()  [unwired: 2 in, 2 out]
                n1768 = property on="SELECT LAB01-2" class="RadioBtnsControl (strict)"("DisabledEnum"=w3335) -> ()  [unwired: 2 in, 2 out]
                n1769 = Not(x=w3345) -> (.not. x?=w3346:bool)
                n1770 = property on="RESULT LAB01-1" class="Bool (strict)"("Visible"=w3346) -> ()  [unwired: 2 in, 2 out]
                n1771 = Not(x=w3340) -> (.not. x?=w3344:bool)
                n1772 = Not(x=w3339) -> (.not. x?=w3343:bool)
                n1773 = Not(x=w3337) -> (.not. x?=w3342:bool)
                n1774 = property on="RESULT LAB01-2" class="Bool (strict)"("Visible"=w3344) -> ()  [unwired: 2 in, 2 out]
                n1775 = Not(x=w3338) -> (.not. x?=w3341:bool)
                n1776 = property on="RESULT LAB02-1" class="Bool (strict)"("Visible"=w3343) -> ()  [unwired: 2 in, 2 out]
                n1777 = property on="RESULT LAB02-2" class="Bool (strict)"("Visible"=w3342) -> ()  [unwired: 2 in, 2 out]
                n1778 = property on="RESULT LAB03-1" class="Bool (strict)"("Visible"=w3341) -> ()  [unwired: 2 in, 2 out]
                n1779 = property on="SET LAB01-1" class="Clust (strict)"("DisabledEnum"=w3336) -> ()  [unwired: 2 in, 2 out]
                n1780 = property on="SET LAB01-2" class="Clust (strict)"("DisabledEnum"=w3335) -> ()  [unwired: 2 in, 2 out]
                n1781 = property on="SET LAB02-1" class="Clust (strict)"("DisabledEnum"=w3334) -> ()  [unwired: 2 in, 2 out]
                n1782 = property on="SET LAB02-2" class="Clust (strict)"("DisabledEnum"=w3333) -> ()  [unwired: 2 in, 2 out]
